vi "FeedbackDecode_GenContTarget.vi"(4 "Gain":dbl=1.0 min=-1.0 max=1.0, 5 "StepTime (ms)":dbl=1000.0 min=0.0, 6 "MvntClust":T1={"MvntMat"=[], "MvntName"="", "Tracking"=enum."False", "Radius"=0.15} {"Radius" min=0.0 max=1.0 step=0.01}, 7 "LoopPeriod (ms)":u64=10 caption="Loop Period (ms)", 8 "LoopCount":dbl, 9 "Mode":enum16{"Initialize", "Reset", "Run"}(ring)) -> (0 "ContSphereVal":dbl[][](array[numeric]), 1 "ContTargetVal":dbl[](array[numeric]), 2 "MaxTimes (ms)":T2, 3 "State":enum16{"Running", "Finished"}(ring)=enum."Finished")   [LabVIEW 2020]
uses:
  <vilib>/Analysis/NI_AALBase.lvlib
panel:
  out "ZeroTargetVal":dbl[](array[numeric])
  out "ZeroSphereVal":dbl[][](array[numeric])
  out "ContTargetArray":dbl[][](array[numeric])
  out "BaseCount":dbl
  # "Thumb"
  # "Index"
  # "Middle"
  # "Ring"
  # "Little"
  # "ThumbInt"
  # "IndexInt"
  # "RingInt"
  # "LittleInt"
  # "WristPitch"
  # "WristYaw"
  # "WristRoll"
  # "Amp"
  # "Del"
  # "Rise"
  # "Hold"
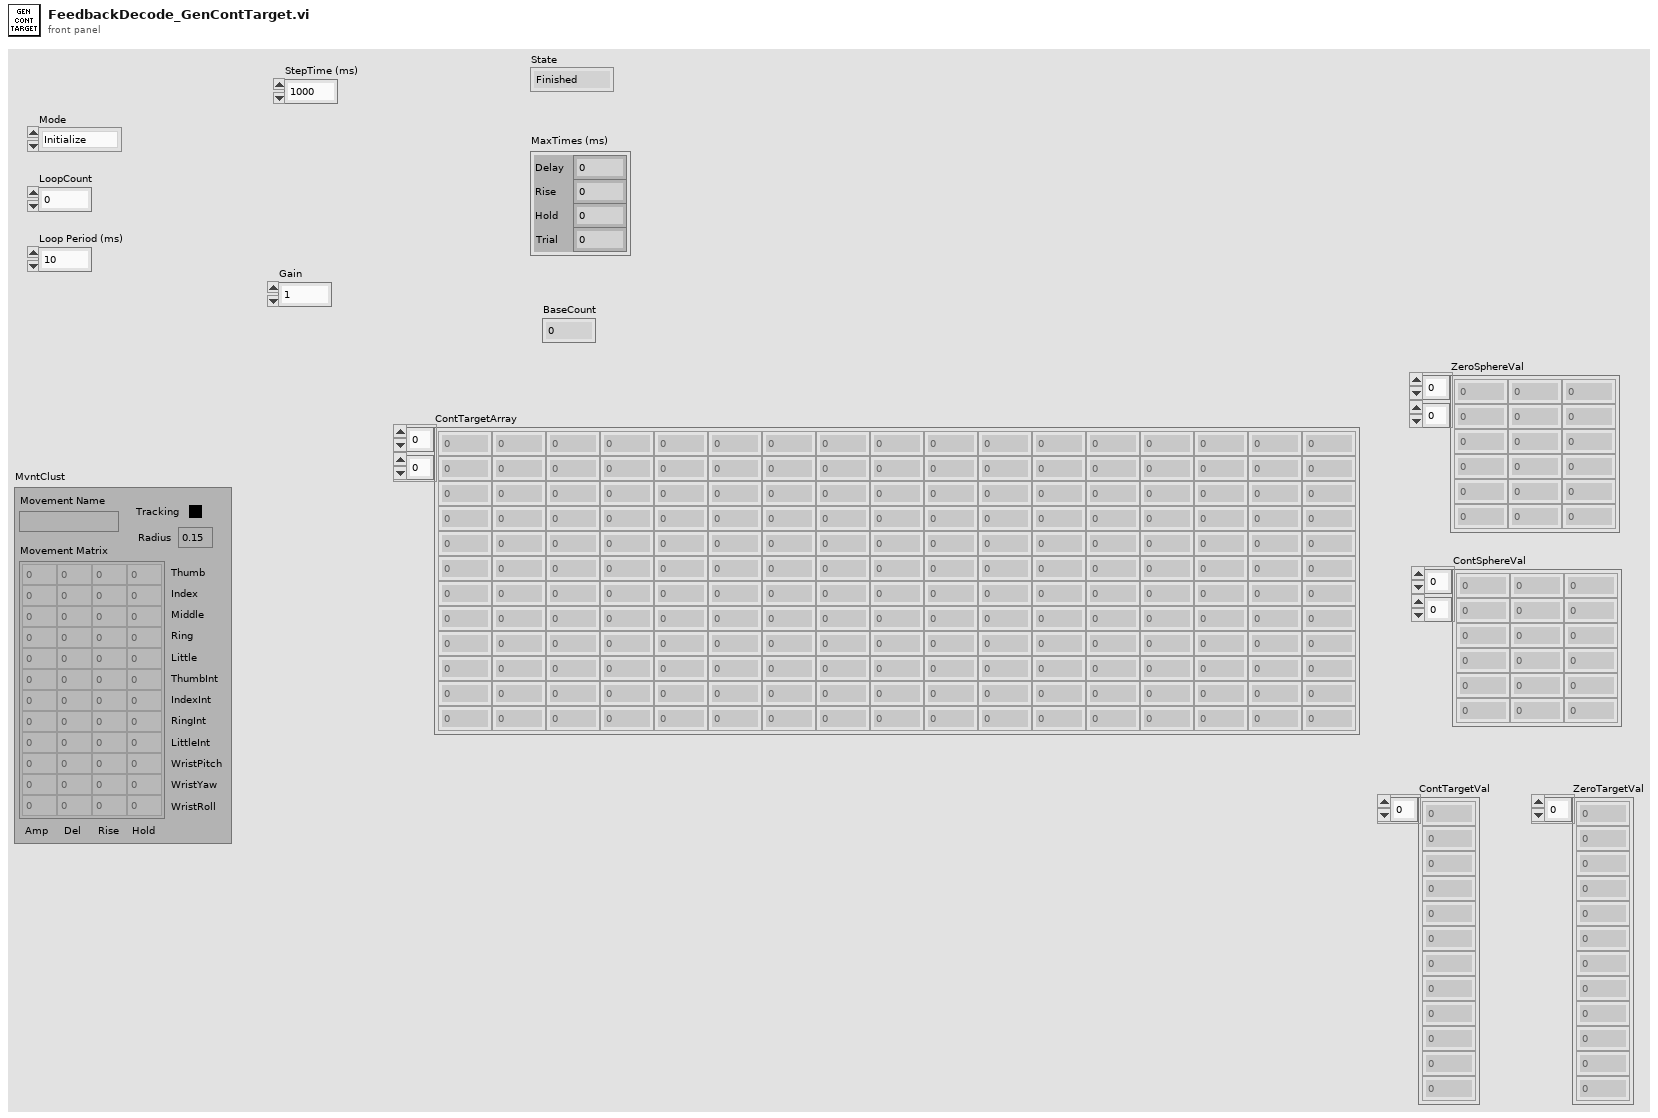
[diagram p1: front panel]
types:
  T1 = cluster{"MvntMat":dbl[][], "MvntName":string, "Tracking":enum8{"False", "True", "Mixed"}, "Radius":dbl}
  T2 = cluster{"Delay":dbl, "Rise":dbl, "Hold":dbl, "Trial":dbl}
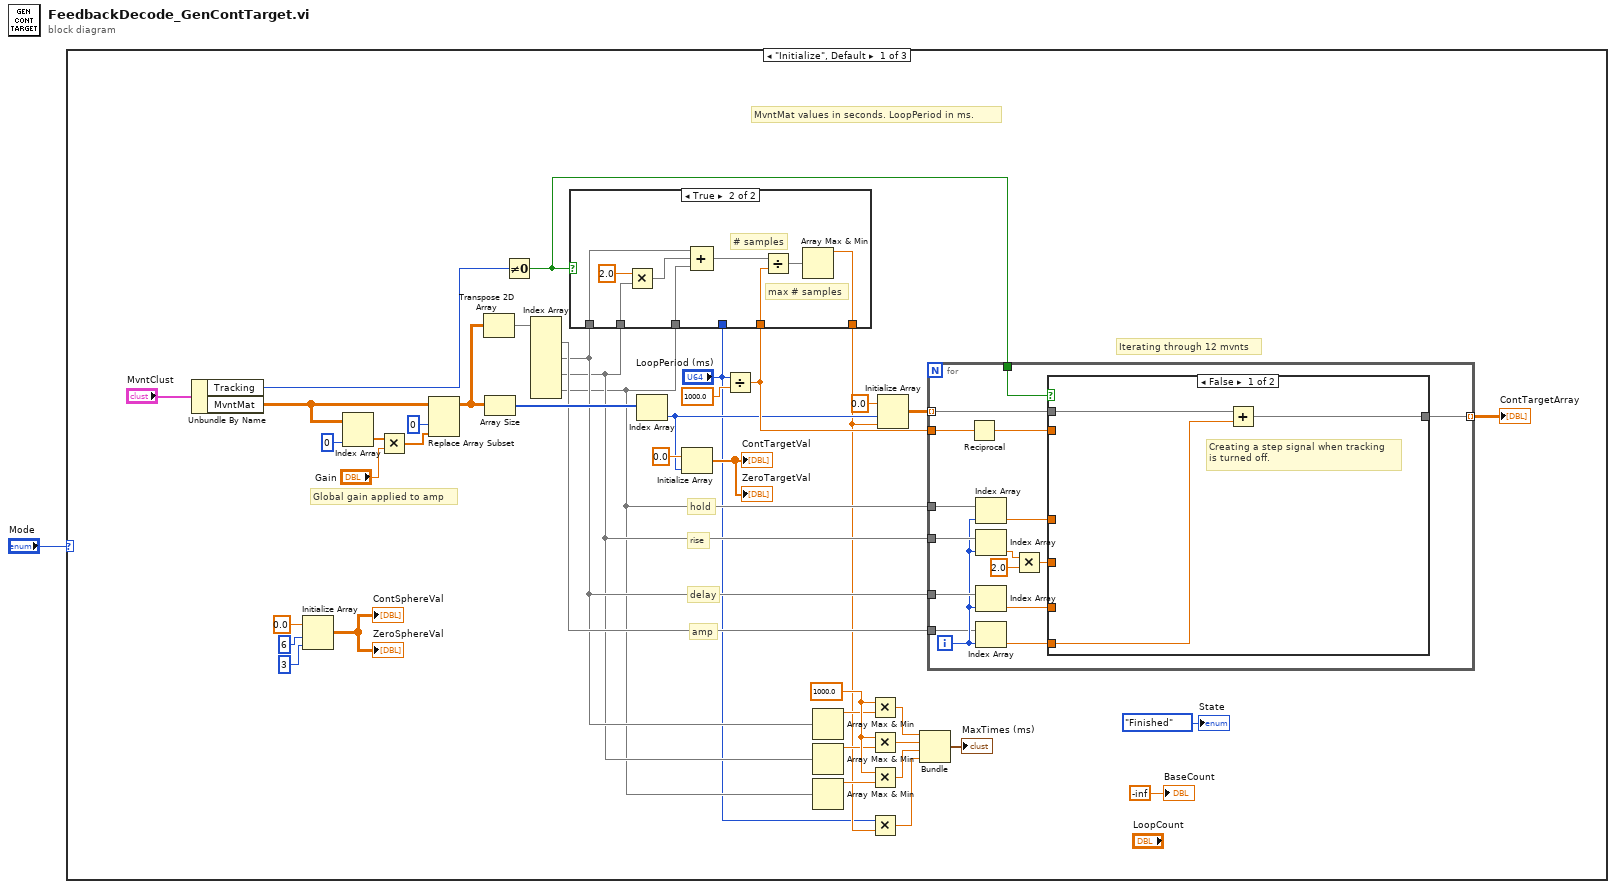
[diagram p0: block diagram]
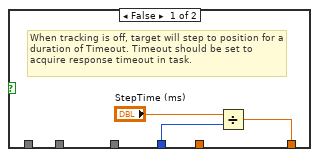
[diagram p2: hidden frame]
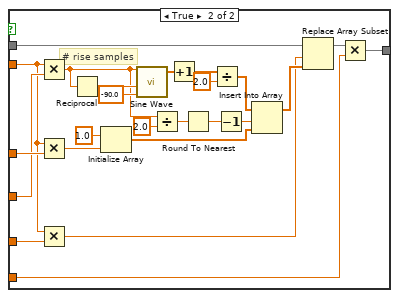
[diagram p3: hidden frame]
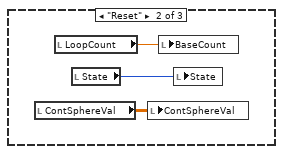
[diagram p4: hidden frame]
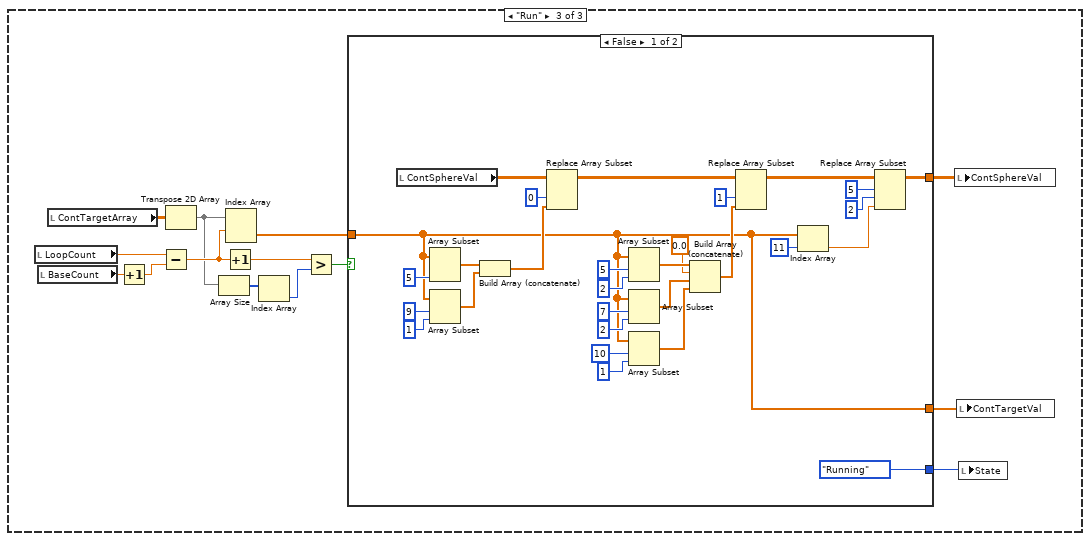
[diagram p5: hidden frame]
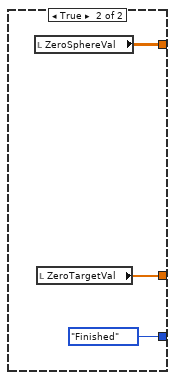
[diagram p6: hidden frame]
diagram:
  n1 = case shown="\"Initialize\", Default" "Mode" {
    frame "Initialize", Default {
      w12 = 1000.0 ("x")
      # "Global gain applied to amp"
      # "Iterating through 12 mvnts"
      # "amp"
      # "MvntMat values in seconds. LoopPeriod in ms."
      # "hold"
      # "rise"
      # "delay"
      n2 = Unbundle By Name("MvntClust") -> ("Tracking"=w19:enum8{"False", "True", "Mixed"}, "MvntMat"=w22:dbl[][])
      n3 = Initialize Array(0.0 ("element"), 6 ("dimension size"), 3 ("dimension size")) -> (→"ContSphereVal" →"ZeroSphereVal":dbl[][])
      n4 = Index Array(array=w22, index (col)=0 ("disabled index (col)")) -> (element=w23:dbl[])  [unwired: 1 in]
      n5 = Multiply(x=w23, y="Gain") -> (x*y=w25:dbl[])
      n6 = Replace Array Subset(array=w22, new element=w25, index (col)=0 ("disabled index (col)")) -> (w21:dbl[][])  [unwired: 1 in]
      n7 = Transpose 2D Array(2D array=w21) -> (transposed array=w39:dbl[][])
      n8 = Array Size(array=w21) -> (size(s)=w38:i32[])
      n9 = Not Equal To 0?(x=w19) -> (x != 0?=w18:bool)
      n10 = Index Array(array=w39) -> (element #1=w32:dbl[], element #2=w8:dbl[], element #3=w7:dbl[], element #4=w6:dbl[])  [unwired: 8 in]
      n11 = Index Array(array=w38) -> (element=w28:i32)  [unwired: 1 in]
      n12 = Initialize Array(0.0 ("element"), w28) -> (→"ZeroTargetVal" →"ContTargetVal":dbl[])
      n13 = Divide(x="LoopPeriod (ms)", y=1000.0) -> (x/y=w35:dbl)
      n14 = case shown="True" w18 {
        tunnel: [w43 w54] -> w5
        tunnel: w8 -> [_ w49]
        tunnel: w7 -> [_ w48]
        tunnel: w6 -> [_ w47]
        tunnel: w35 -> [_ w46]
        tunnel: "LoopPeriod (ms)" -> [w44 _]
        frame False {
          # "When tracking is off, target will step to position for a duration of Timeout. Timeout should be set to acquire response timeout in task."
          n15 = Divide(x="StepTime (ms)", y=w44) -> (x/y=w43:dbl)
        }
        frame True {
          # "max # samples"
          # "# samples"
          n16 = Multiply(x=2.0, y=w48) -> (x*y=w51:dbl[])
          n17 = Compound Arithmetic op=ADD(w49, w51, w47) -> (w52:dbl[])
          n18 = Divide(x=w52, y=w46) -> (x/y=w53:dbl[])
          n19 = Array Max & Min(array=w53) -> (max value=w54:dbl)  [unwired: 3 out]
        }
      }
      n20 = Array Max & Min(array=w8) -> (max value=w11:dbl)  [unwired: 3 out]
      n21 = Array Max & Min(array=w7) -> (max value=w10:dbl)  [unwired: 3 out]
      n22 = Array Max & Min(array=w6) -> (max value=w9:dbl)  [unwired: 3 out]
      n23 = Multiply(x=w12, y=w11) -> (x*y=w13:dbl)
      n24 = Multiply(x=w12, y=w10) -> (x*y=w14:dbl)
      n25 = Multiply(x=w12, y=w9) -> (x*y=w15:dbl)
      n26 = Multiply(x="LoopPeriod (ms)", y=w5) -> (x*y=w17:dbl)
      n27 = Initialize Array(0.0, w28, w5) -> (w37:dbl[][])
      n28 = Bundle(w13, w14, w15, w17) -> (→"MaxTimes (ms)":cluster{dbl, dbl, dbl, dbl})  [unwired: 1 in]
      n29 = for {
        tunnel: w37 -> [w66] mode=indexing
        tunnel: w8 -> [w70]
        tunnel: w7 -> [w69]
        tunnel: w6 -> [w68]
        tunnel: w35 -> [w65]
        tunnel: [w57] -> w34 mode=indexing
        tunnel: w32 -> [w58]
        tunnel: w18 -> [w56]
        i -> [w59]
        n30 = Reciprocal(x=w65) -> (1/x=w61:dbl)
        n31 = Index Array(array=w68, index=w59) -> (element=w67:dbl)
        n32 = Index Array(array=w69, index=w59) -> (element=w64:dbl)
        n33 = Index Array(array=w70, index=w59) -> (element=w60:dbl)
        n34 = Index Array(array=w58, index=w59) -> (element=w55:dbl)
        n35 = Multiply(x=w64, y=2.0) -> (x*y=w62:dbl)
        n36 = case shown="False" w56 {
          tunnel: w67 -> [_ w83]
          tunnel: w66 -> [w73 w82]
          tunnel: w62 -> [_ w80]
          tunnel: w61 -> [_ w79]
          tunnel: w60 -> [_ w78]
          tunnel: [w71 w76] -> w57
          tunnel: w55 -> [w72 w74]
          frame False {
            # "Creating a step signal when tracking\nis turned off."
            n37 = Add(x=w73, y=w72) -> (x+y=w71:dbl[])
          }
          frame True {
            # "# rise samples"
            n38 = Multiply(x=w79, y=w80) -> (x*y=w88:dbl)
            n39 = Multiply(x=w79, y=w83) -> (x*y=w92:dbl)
            n40 = Multiply(x=w79, y=w78) -> (x*y=w75:dbl)
            n41 = Reciprocal(x=w88) -> (1/x=w97:dbl)
            n42 = Initialize Array(1.0, w92) -> (w84:dbl[])
            n43 = call <vilib>:"Sine Wave.vi"("samples"=w88, "frequency"=w97, "phase in"=-90.0) -> ("sine wave"=w95:dbl[])  [unwired: 2 in, 2 out]
            n44 = Divide(x=w88, y=2.0) -> (x/y=w87:dbl)
            n45 = Increment(x=w95) -> (x+1=w94:dbl[])
            n46 = Round To Nearest(number=w87) -> (nearest integer value=w86:dbl)
            n47 = Divide(x=w94, y=2.0) -> (x/y=w90:dbl[])
            n48 = Decrement(x=w86) -> (x-1=w85:dbl)
            n49 = Insert Into Array(array=w90, index=w85, new element=w84) -> (w81:dbl[])
            n50 = Replace Array Subset(array=w82, new element=w81, index=w75) -> (w77:dbl[])
            n51 = Multiply(x=w77, y=w74) -> (x*y=w76:dbl[])
          }
        }
      }
      "ContTargetArray" <- w34
      "BaseCount" <- -inf
      "State" <- enum16{"Running", "Finished"}."Finished" ("State")
    }
    frame "Reset" {
      n52 = local read "ContSphereVal"() -> (w98:dbl[][])
      n53 = local read "LoopCount"() -> (w100:dbl)
      n54 = local read "State"() -> (w99:enum16{"Running", "Finished"})
      n55 = local write "ContSphereVal"(w98) -> ()
      n56 = local write "BaseCount"(w100) -> ()
      n57 = local write "State"(w99) -> ()
    }
    frame "Run" {
      n58 = local read "LoopCount"() -> (w113:dbl)
      n59 = local read "BaseCount"() -> (w114:dbl)
      n60 = local read "ContTargetArray"() -> (w107:dbl[][])
      n61 = Increment(x=w114) -> (x+1=w112:dbl)
      n62 = Subtract(x=w113, y=w112) -> (x-y=w106:dbl)
      n63 = Transpose 2D Array(2D array=w107) -> (transposed array=w105:dbl[][])
      n64 = Array Size(array=w105) -> (size(s)=w104:i32[])
      n65 = Increment(x=w106) -> (x+1=w111:dbl)
      n66 = Index Array(array=w105, index (row)=w106) -> (element=w109:dbl[])  [unwired: 1 in]
      n67 = Index Array(array=w104) -> (element=w103:i32)  [unwired: 1 in]
      n68 = Greater?(x=w111, y=w103) -> (0:w110:bool)
      n69 = case shown="False" w110 {
        tunnel: w109 -> [w115 _]
        tunnel: [w119 w145] -> w102
        tunnel: [enum16{"Running", "Finished"}."Running" ("State") enum16{"Running", "Finished"}."Finished" ("State")] -> w108
        tunnel: [w115 w144] -> w101
        frame False {
          n70 = local read "ContSphereVal"() -> (w142:dbl[][])
          n71 = Array Subset(array=w115, length=5) -> (w138:dbl[])  [unwired: 1 in]
          n72 = Array Subset(array=w115, index=9, length=1) -> (w137:dbl[])
          n73 = Build Array (concatenate)(w138, w137) -> (w135:dbl[])
          n74 = Replace Array Subset(array=w142, new element=w135, index (col)=0 ("disabled index (col)")) -> (w130:dbl[][])  [unwired: 1 in]
          n75 = Array Subset(array=w115, index=5, length=2) -> (w128:dbl[])
          n76 = Array Subset(array=w115, index=7, length=2) -> (w124:dbl[])
          n77 = Array Subset(array=w115, index=10, length=1) -> (w123:dbl[])
          n78 = Build Array (concatenate)(w128, 0.0, w124, w123) -> (w122:dbl[])
          n79 = Replace Array Subset(array=w130, new element=w122, index (col)=1 ("disabled index (col)")) -> (w120:dbl[][])  [unwired: 1 in]
          n80 = Index Array(array=w115, index=11) -> (element=w116:dbl)
          n81 = Replace Array Subset(array=w120, new element=w116, index (row)=5 ("disabled index (row)"), index (col)=2 ("disabled index (col)")) -> (w119:dbl[][])
        }
        frame True {
          n82 = local read "ZeroSphereVal"() -> (w145:dbl[][])
          n83 = local read "ZeroTargetVal"() -> (w144:dbl[])
        }
      }
      n84 = local write "ContSphereVal"(w102) -> ()
      n85 = local write "ContTargetVal"(w101) -> ()
      n86 = local write "State"(w108) -> ()
    }
  }
